vi "Li_Query_and_write_svi.vi"(8 "error in (no error)":errorcluster, 11 "Key Index":i32) -> (0 "error out":errorcluster, 2 "Numeric":i32, 3 "OUT":i32)   [LabVIEW 2015]
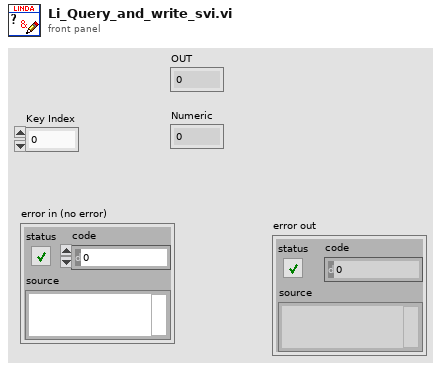
[diagram p1: front panel]
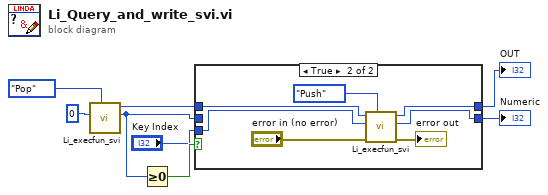
[diagram p0: block diagram]
diagram:
  n1 = call "Li_execfun_svi.vi"("OP"=enum16{"INIT", "Push", "Pop", "Query"}."Pop", "Key Index"=0) -> ("Size"=w1:i32, "Addr"=w2:i32)  [unwired: 7 in, 1 out]
  n2 = Greater Or Equal To 0?(x=w1) -> (x >= 0?=w8:bool)
  n3 = case shown="True" w8 {
    tunnel: w2 -> [_ w16]
    tunnel: [_ w14] -> w6
    tunnel: [w9 w13] -> w7
    tunnel: w1 -> [w9 _]
    tunnel: "Key Index" -> [_ w12]
    frame False {
      # "Failed because no free space"
    }
    frame True {
      n4 = call "Li_execfun_svi.vi"("OP"=enum16{"INIT", "Push", "Pop", "Query"}."Push", "error in (no error)"="error in (no error)", "Key Index"=w12, "IN"=w16) -> ("error out"=→"error out":errorcluster, "Size"=w13:i32, "Addr"=w14:i32)  [unwired: 5 in]
    }
  }
  "Numeric" <- w7
  "OUT" <- w6
